vi "DAC Save Results.vi"(8 "error in":errorcluster, 9 "Log Details?":bool, 10 "tdms file":refnum<k34>, 11 "DAC HeatFlow AOV in":refnum<class "DAC HeatFlow AOV.lvclass">) -> (0 "error out":errorcluster)   [LabVIEW 2019, in "DAC.lvlib" / "DAC HeatFlow AOV.lvclass"]
uses:
  DAC HeatFlow AOV.lvclass
  DAC.lvclass
  C:/Users/wg/Documents/LV_Projects/test-stand/App/DAC/DAC.lvclass
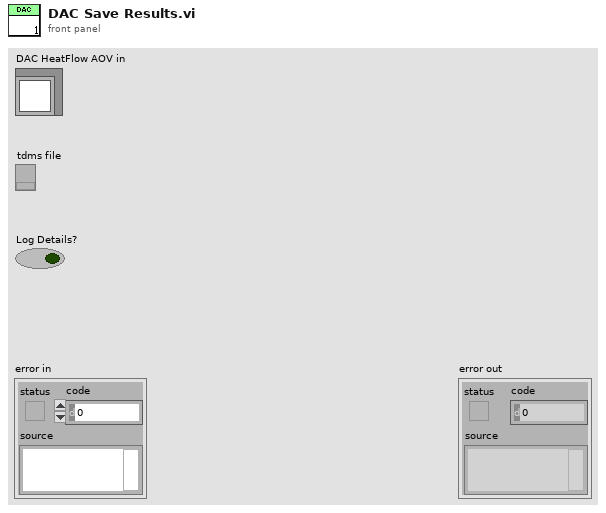
[diagram p1: front panel]
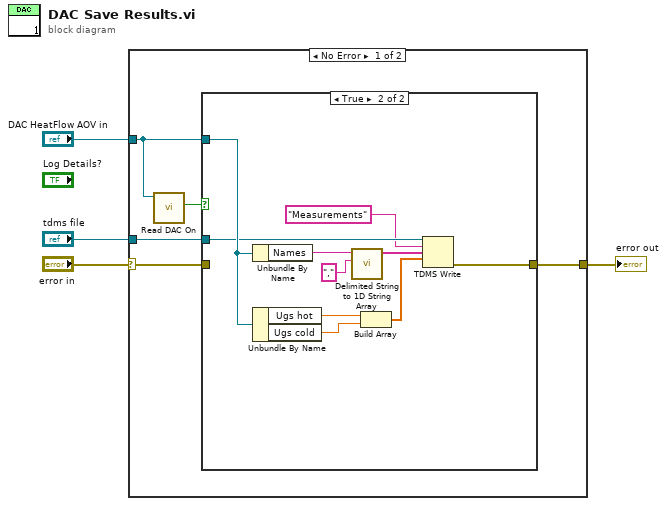
[diagram p0: block diagram]
diagram:
  n1 = case shown="No Error" "error in" {
    selector: "error in" -> [w6 w21]
    tunnel: "DAC HeatFlow AOV in" -> [w9 _]
    tunnel: "tdms file" -> [w7 _]
    tunnel: [w5 w21] -> w1
    frame No Error {
      n2 = call "Read DAC On.vi"("DAC in"=w9) -> ("DAC On"=w8:bool)  [unwired: 8 in, 2 out]
      n3 = case shown="True" w8 {
        tunnel: w9 -> [_ w20]
        tunnel: w7 -> [_ w12]
        tunnel: w6 -> [w10 _]
        tunnel: [w10 w13] -> w5
        frame False {
        }
        frame True {
          n4 = Unbundle By Name(w20) -> ("Names"=w18:string)
          n5 = Unbundle By Name(w20) -> ("Ugs hot"=w16:dbl, "Ugs cold"=w15:dbl)
          n6 = call <vilib>:"Delimited String to 1D String Array.vi"("delimiter"=",", "delimited string"=w18) -> ("string array"=w17:string[])  [unwired: 9 in]
          n7 = Build Array(w16, w15) -> (w14:dbl[])
          n8 = TDMS Write(0:w12, 5:"Measurements" ("group name in (Untitled)"), 7:w17, 9:w14) -> (15:w13:errorcluster)  [unwired: 2 in, 3 out]
        }
      }
    }
    frame Error {
    }
  }
  "error out" <- w1
